vi "FTW-JSON-Core-GetFlattenedValue.vi"(0 "Library Filepath":path, 5 "JSON Element":i64 format="%016x", 7 "LabVIEW Type":T1, 9 "Element Default Value":variant, 11 "error in":errorcluster, 12 "Encoding Flags":i64 format="%016x") -> (4 "Flattened Value":string, 15 "error out":errorcluster)   [LabVIEW 2014, in "FTW-JSON-Fetch.xnode"]
uses:
  FTW-JSON-Fetch.xnode
  src/reflection/FTW-Reflection-Types.ctl
  src/json/core/FTW-JSON-Core-Type.ctl
  src/error/FTW-ERR-ThrowError.vi
  src/error/FTW-ERR-NoErrorConstant.vi
  src/error/FTW-ERR-CallChain.vi
  src/string/FTW-STR-ReplaceWhitespace.vi
panel:
  # "Inputs"
  # "Outputs"
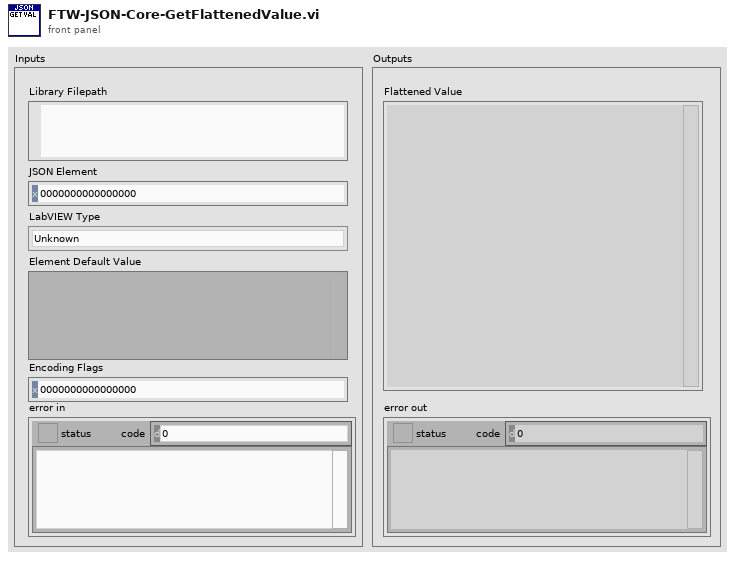
[diagram p1: front panel]
types:
  T1 = typedef "FTW-Reflection-Types.ctl" = enum16{"Unknown", "Void", "Array", "Cluster", "LVObject", "Boolean", "I8", "I16", "I32", "I64", "U8", "U16", "U32", "U64", "SGL", "DBL", "EXT", "CSG", "CDB", "CXT", "FXP", "EnumU8", "EnumU16", "EnumU32", "EnumU64", "SGLwithUnit", "DBLwithUnit", "EXTwithUnit", "CSGwithUnit", "CDBwithUnit", "CXTwithUnit", "String", "Path", "Picture", "Tag", "LVVariant", "Timestamp", "WaveformI8", "WaveformI16", "WaveformI32", "WaveformI64", "WaveformU8", "WaveformU16", "WaveformU32", "WaveformU64", "WaveformSGL", "WaveformDBL", "WaveformEXT", "WaveformCSG", "WaveformCDB", "WaveformCXT", "WaveformDigital", "WaveformUnknownType", "DigitalData", "DynamicData", "ExternalData", "FileByteStream", "TDMStream", "dotNET", "ActiveX", "VIServerReference", "VIReference", "ApplicationInstance", "Menu", "ConnectionDataSocket", "ConnectionVISA", "ConnectionBluetooth", "ConnectionIrDA", "ConnectionTCP", "ConnectionUDP", "ConnectionHTTPClient", "ConnectionFTP", "Occurrence", "Notifier", "Queue", "Rendezvous", "Semaphore", "RTFIFO", "EventPublisher", "EventRegistration", "EventCallback", "DataValueReference", "GenericClass", "GenericClassTag", "GenericClassDeepCopy", "GenericClassFlattened", "GenericClassTagFlattened", "GenericReferenceType", "WindowsRegistry", "OverloadedDatalogRef", "ReferenceUnknownType", "ByteArray"}
  T2 = typedef "FTW-JSON-Core-Type.ctl" = enum8{"Object", "Array", "String", "Integer", "Floating Point", "true", "false", "null", "undefined"}
  T3 = cluster{"Element Name":string, "Element Type":T1, "Element Value":variant}[]
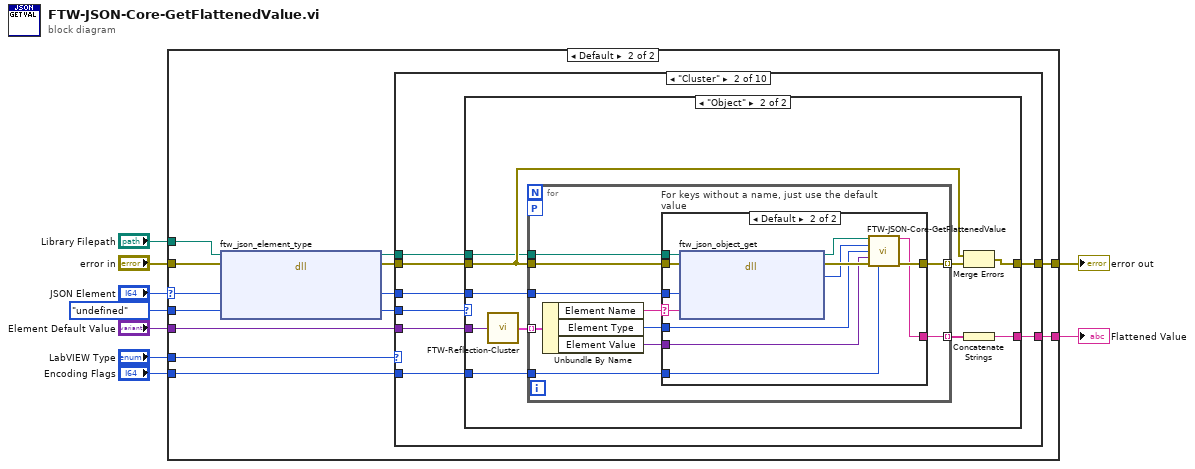
[diagram p0: block diagram]
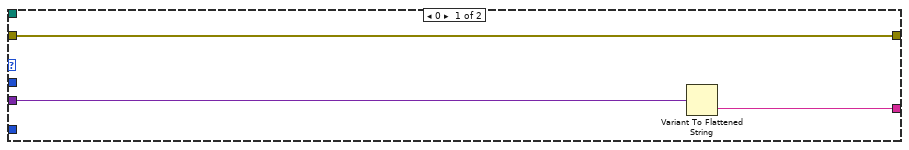
[diagram p2: hidden frame]
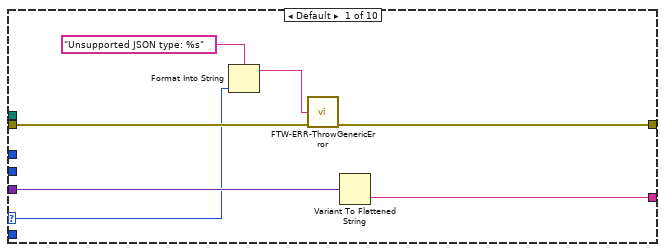
[diagram p3: hidden frame]
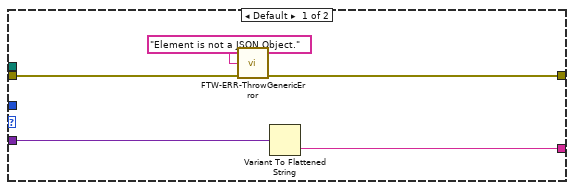
[diagram p4: hidden frame]
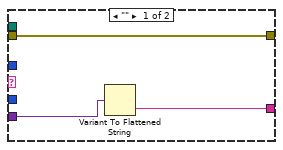
[diagram p5: hidden frame]
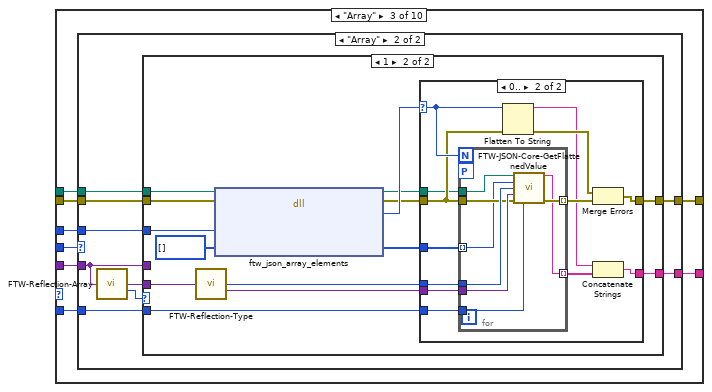
[diagram p6: hidden frame]
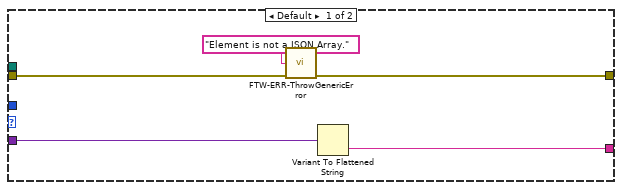
[diagram p7: hidden frame]
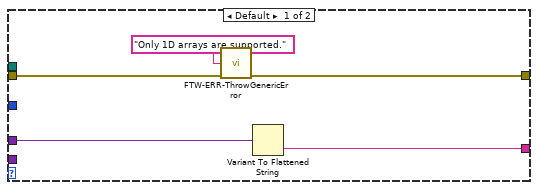
[diagram p8: hidden frame]
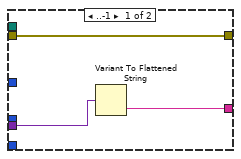
[diagram p9: hidden frame]
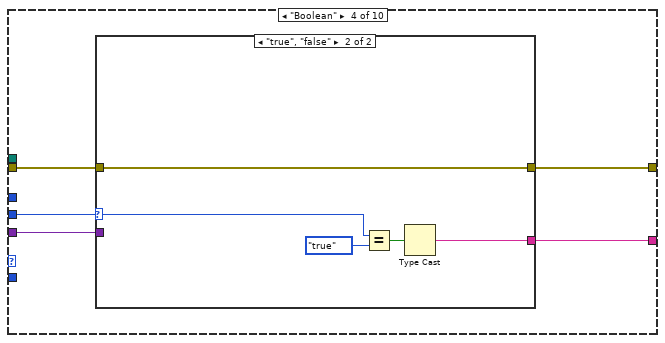
[diagram p10: hidden frame]
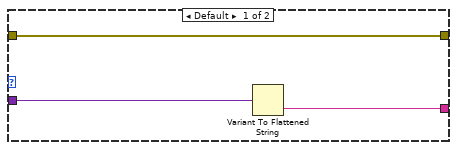
[diagram p11: hidden frame]
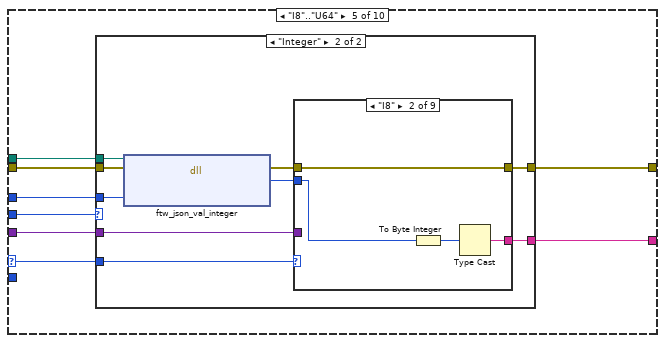
[diagram p12: hidden frame]
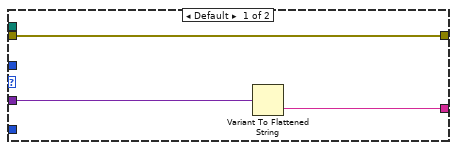
[diagram p13: hidden frame]
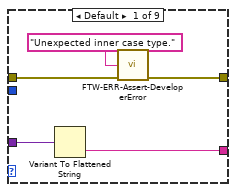
[diagram p14: hidden frame]
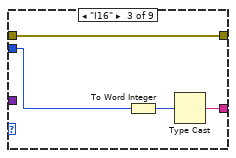
[diagram p15: hidden frame]
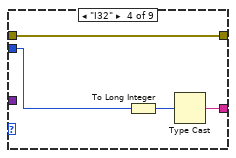
[diagram p16: hidden frame]
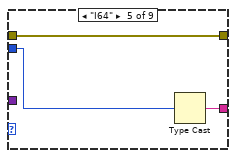
[diagram p17: hidden frame]
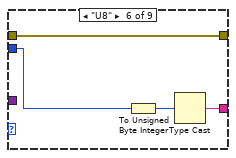
[diagram p18: hidden frame]
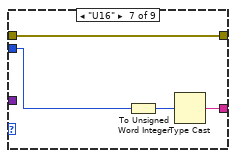
[diagram p19: hidden frame]
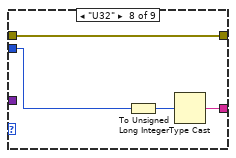
[diagram p20: hidden frame]
diagram:
  n1 = case shown="Default" "JSON Element" {
    selector: "JSON Element" -> [_ w20]
    tunnel: [w10 w25] -> w9
    tunnel: [w11 w24] -> w7
    tunnel: "LabVIEW Type" -> [_ w23]
    tunnel: "Element Default Value" -> [w12 w22]
    tunnel: "error in" -> [w10 w14]
    tunnel: "Encoding Flags" -> [_ w21]
    tunnel: FTW-JSON-Core-Type."undefined" ("x") -> [_ w18]
    tunnel: "Library Filepath" -> [_ w15]
    frame 0 {
      n2 = Variant To Flattened String(Variant=w12) -> (data string=w11:string)  [unwired: 1 out]
    }
    frame Default {
      n3 = dll-call lib="?" fn="ftw_json_element_type"(path in=w15, error in=w14, "JSON Element"=w20, "JSON Type"=w18) -> (path out=w13:path, error out=w16:errorcluster, "JSON Element"=w19:i64, "JSON Type"=w17:T2)  [unwired: 2 in]
      n4 = case shown="\"Cluster\"" w23 {
        selector: w23 -> [w26 _ _ _ w163 w219 w303 _ w379 _]
        tunnel: [w29 w37 w86 w146 w160 w216 w300 w358 w376 w428] -> w25
        tunnel: [w27 w39 w87 w149 w165 w221 w305 w362 w381 w432] -> w24
        tunnel: w16 -> [w30 w36 w85 w150 w166 w222 w306 w363 w382 w433]
        tunnel: w19 -> [_ w38 w83 _ w162 w218 w302 w360 w378 w430]
        tunnel: w22 -> [w28 w40 w88 w148 w164 w220 w304 w361 w380 w431]
        tunnel: w17 -> [_ w35 w84 w147 w161 w217 w301 w359 w377 w429]
        tunnel: w21 -> [_ w34 w82 _ _ _ _ _ w375 _]
        tunnel: w13 -> [_ w33 w81 _ w159 w215 w299 w357 w374 w427]
        frame Default {
          n5 = Format Into String(format string="Unsupported JSON type: %s", w26) -> (resulting string=w32:string)  [unwired: 2 in, 1 out]
          n6 = call "FTW-ERR-ThrowGenericError.vi"("Error Message"=w32, "error in"=w30) -> ("error out"=w29:errorcluster)  [unwired: 13 in]
          n7 = Variant To Flattened String(Variant=w28) -> (data string=w27:string)  [unwired: 1 out]
        }
        frame "Cluster" {
          n8 = case shown="\"Object\"" w35 {
            tunnel: w40 -> [w43 w55]
            tunnel: [w42 w54] -> w39
            tunnel: w38 -> [_ w47]
            tunnel: [w44 w53] -> w37
            tunnel: w36 -> [w45 w48]
            tunnel: w34 -> [_ w52]
            tunnel: w33 -> [_ w46]
            frame Default {
              n9 = call "FTW-ERR-ThrowGenericError.vi"("Error Message"="Element is not a JSON Object.", "error in"=w45) -> ("error out"=w44:errorcluster)  [unwired: 13 in]
              n10 = Variant To Flattened String(Variant=w43) -> (data string=w42:string)  [unwired: 1 out]
            }
            frame "Object" {
              n11 = call "FTW-Reflection-Cluster.vi"("Cluster"=w55) -> ("Cluster Elements"=w51:T3)  [unwired: 14 in]
              n12 = for {
                tunnel: w51 -> [w64] mode=indexing
                tunnel: [w62] -> w50 mode=indexing
                tunnel: w47 -> [w59]
                tunnel: w48 -> [w65]
                tunnel: [w60] -> w49 mode=indexing
                workers-P: _ -> [_]
                tunnel: w52 -> [w58]
                tunnel: w46 -> [w56]
                n13 = Unbundle By Name(w64) -> ("Element Name"=w57:string, "Element Type"=w61:T1, "Element Value"=w63:variant)
                n14 = case "For keys without a name, just use the default value" shown="Default" w57 {
                  selector: w57 -> [_ w77]
                  tunnel: w65 -> [w66 w79]
                  tunnel: w63 -> [w68 w74]
                  tunnel: [w67 w75] -> w62
                  tunnel: w59 -> [_ w78]
                  tunnel: w61 -> [_ w73]
                  tunnel: [w66 w76] -> w60
                  tunnel: w58 -> [_ w71]
                  tunnel: w56 -> [_ w70]
                  frame "" {
                    n15 = Variant To Flattened String(Variant=w68) -> (data string=w67:string)  [unwired: 1 out]
                  }
                  frame Default {
                    n16 = dll-call lib="?" fn="ftw_json_object_get"(path in=w70, error in=w79, "JSON Object Pointer"=w78, "Element Key"=w77) -> (path out=w69:path, error out=w80:errorcluster, "JSON Element Pointer"=w72:i64)  [unwired: 3 in]
                    n17 = call "FTW-JSON-Core-GetFlattenedValue.vi"("Library Filepath"=w69, "JSON Element"=w72, "LabVIEW Type"=w73, "Element Default Value"=w74, "error in"=w80, "Encoding Flags"=w71) -> ("Flattened Value"=w75:string, "error out"=w76:errorcluster)  [unwired: 8 in]
                  }
                }
              }
              n18 = Merge Errors(w48, w49) -> (w53:errorcluster)
              n19 = Concatenate Strings(w50) -> (w54:string)
            }
          }
        }
        frame "Array" {
          n20 = case shown="\"Array\"" w84 {
            tunnel: w88 -> [w91 w96]
            tunnel: [w90 w102] -> w87
            tunnel: [w89 w101] -> w86
            tunnel: w85 -> [w92 w100]
            tunnel: w83 -> [_ w97]
            tunnel: w82 -> [_ w95]
            tunnel: w81 -> [_ w94]
            frame Default {
              n21 = call "FTW-ERR-ThrowGenericError.vi"("Error Message"="Element is not a JSON Array.", "error in"=w92) -> ("error out"=w89:errorcluster)  [unwired: 13 in]
              n22 = Variant To Flattened String(Variant=w91) -> (data string=w90:string)  [unwired: 1 out]
            }
            frame "Array" {
              n23 = call "FTW-Reflection-Array.vi"("Array"=w96) -> ("Default Array Element"=w99:variant, "Number of Dimensions"=w98:i32)  [unwired: 13 in]
              n24 = case shown="1" w98 {
                tunnel: [w104 w121] -> w102
                tunnel: [w105 w120] -> w101
                tunnel: w100 -> [w106 w114]
                tunnel: w99 -> [_ w119]
                tunnel: w97 -> [_ w113]
                tunnel: w96 -> [w103 _]
                tunnel: w95 -> [_ w116]
                tunnel: w94 -> [_ w109]
                frame Default {
                  n25 = call "FTW-ERR-ThrowGenericError.vi"("Error Message"="Only 1D arrays are supported.", "error in"=w106) -> ("error out"=w105:errorcluster)  [unwired: 13 in]
                  n26 = Variant To Flattened String(Variant=w103) -> (data string=w104:string)  [unwired: 1 out]
                }
                frame 1 {
                  n27 = call "FTW-Reflection-Type.vi"("Anything"=w119) -> ("LabVIEW Type"=w118:T1, "Variant Type and Value"=w117:variant)  [unwired: 12 in, 1 out]
                  n28 = dll-call lib="?" fn="ftw_json_array_elements"(path in=w109, error in=w114, "Array Pointer"=w113, "Items"=i64[] []) -> (path out=w108:path, error out=w110:errorcluster, "Elements"=w112:i32, "Items"=w111:i64[])  [unwired: 2 in]
                  n29 = case shown="0.." w112 {
                    selector: w112 -> [_ w131]
                    tunnel: [w124 w137] -> w121
                    tunnel: [w122 w136] -> w120
                    tunnel: w110 -> [w122 w128]
                    tunnel: w118 -> [_ w134]
                    tunnel: w117 -> [w123 w133]
                    tunnel: w116 -> [_ w127]
                    tunnel: w111 -> [_ w126]
                    tunnel: w108 -> [_ w125]
                    frame ..-1 {
                      n30 = Variant To Flattened String(Variant=w123) -> (data string=w124:string)  [unwired: 1 out]
                    }
                    frame 0.. {
                      n31 = for {
                        N: w131 -> [_]
                        workers-P: _ -> [_]
                        tunnel: w128 -> [w140]
                        tunnel: [w145] -> w135 mode=indexing
                        tunnel: w134 -> [w142]
                        tunnel: w133 -> [w143]
                        tunnel: [w144] -> w132 mode=indexing
                        tunnel: w127 -> [w141]
                        tunnel: w126 -> [w139] mode=indexing
                        tunnel: w125 -> [w138]
                        n32 = call "FTW-JSON-Core-GetFlattenedValue.vi"("Library Filepath"=w138, "JSON Element"=w139, "LabVIEW Type"=w142, "Element Default Value"=w143, "error in"=w140, "Encoding Flags"=w141) -> ("Flattened Value"=w144:string, "error out"=w145:errorcluster)  [unwired: 8 in]
                      }
                      n33 = Flatten To String(anything=w131, error in (no error)=w128) -> (data string=w129:string, error out=w130:errorcluster)  [unwired: 2 in, 1 out]
                      n34 = Merge Errors(w130, w135) -> (w136:errorcluster)
                      n35 = Concatenate Strings(w129, w132) -> (w137:string)
                    }
                  }
                }
              }
            }
          }
        }
        frame "Boolean" {
          n36 = case shown="\"true\", \"false\"" w147 {
            selector: w147 -> [_ w156]
            tunnel: w150 -> [w151 w157]
            tunnel: w148 -> [w153 _]
            tunnel: [w152 w158] -> w149
            tunnel: [w151 w157] -> w146
            frame Default {
              n37 = Variant To Flattened String(Variant=w153) -> (data string=w152:string)  [unwired: 1 out]
            }
            frame "true", "false" {
              n38 = Equal?(x=w156, y=FTW-JSON-Core-Type."true" ("x")) -> (x = y?=w154:bool)
              n39 = Type Cast(x=w154) -> (*(type *) &x=w158:string)  [unwired: 1 in]
            }
          }
        }
        frame "I8".."U64" {
          n40 = case shown="\"Integer\"" w161 {
            tunnel: w162 -> [_ w178]
            tunnel: w166 -> [w167 w177]
            tunnel: w164 -> [w169 w171]
            tunnel: [w168 w172] -> w165
            tunnel: [w167 w175] -> w160
            tunnel: w163 -> [_ w176]
            tunnel: w159 -> [_ w170]
            frame Default {
              n41 = Variant To Flattened String(Variant=w169) -> (data string=w168:string)  [unwired: 1 out]
            }
            frame "Integer" {
              n42 = dll-call lib="?" fn="ftw_json_val_integer"(path in=w170, error in=w177, "JSON Element Pointer"=w178) -> (error out=w174:errorcluster, "I64 Value"=w173:i64)  [unwired: 2 in, 1 out]
              n43 = case shown="\"I8\"" w176 {
                tunnel: [w182 w187 w191 w195 w198 w202 w206 w210 w214] -> w175
                tunnel: w174 -> [w183 w187 w191 w195 w198 w202 w206 w210 w214]
                tunnel: w173 -> [_ w185 w189 w193 w196 w200 w204 w208 w212]
                tunnel: [w179 w186 w190 w194 w197 w201 w205 w209 w213] -> w172
                tunnel: w171 -> [w180 _ _ _ _ _ _ _ _]
                frame Default {
                  n44 = Variant To Flattened String(Variant=w180) -> (data string=w179:string)  [unwired: 1 out]
                  n45 = call "FTW-ERR-Assert-DeveloperError.vi"("Reason this error should never happen"="Unexpected inner case type.", "error in"=w183) -> ("error out"=w182:errorcluster)  [unwired: 13 in]
                }
                frame "I8" {
                  n46 = To Byte Integer(number=w185) -> (8bit integer=w184:i8)
                  n47 = Type Cast(x=w184) -> (*(type *) &x=w186:string)  [unwired: 1 in]
                }
                frame "I16" {
                  n48 = To Word Integer(number=w189) -> (16bit integer=w188:i16)
                  n49 = Type Cast(x=w188) -> (*(type *) &x=w190:string)  [unwired: 1 in]
                }
                frame "I32" {
                  n50 = To Long Integer(number=w193) -> (32bit integer=w192:i32)
                  n51 = Type Cast(x=w192) -> (*(type *) &x=w194:string)  [unwired: 1 in]
                }
                frame "I64" {
                  n52 = Type Cast(x=w196) -> (*(type *) &x=w197:string)  [unwired: 1 in]
                }
                frame "U8" {
                  n53 = To Unsigned Byte Integer(number=w200) -> (unsigned 8bit integer=w199:u8)
                  n54 = Type Cast(x=w199) -> (*(type *) &x=w201:string)  [unwired: 1 in]
                }
                frame "U16" {
                  n55 = To Unsigned Word Integer(number=w204) -> (unsigned 16bit integer=w203:u16)
                  n56 = Type Cast(x=w203) -> (*(type *) &x=w205:string)  [unwired: 1 in]
                }
                frame "U32" {
                  n57 = To Unsigned Long Integer(number=w208) -> (unsigned 32bit integer=w207:u32)
                  n58 = Type Cast(x=w207) -> (*(type *) &x=w209:string)  [unwired: 1 in]
                }
                frame "U64" {
                  n59 = To Unsigned Quad Integer(1:w212) -> (0:w211:u64)
                  n60 = Type Cast(x=w211) -> (*(type *) &x=w213:string)  [unwired: 1 in]
                }
              }
            }
          }
        }
        frame "EnumU8".."EnumU64" {
          n61 = case shown="\"Integer\"" w217 {
            tunnel: w218 -> [_ w235 w272]
            tunnel: w222 -> [w223 w234 w273]
            tunnel: w220 -> [w225 w229 w277]
            tunnel: [w224 w230 w274] -> w221
            tunnel: [w223 w232 w275] -> w216
            tunnel: w219 -> [_ w233 w276]
            tunnel: w215 -> [_ w226 w269]
            frame Default {
              n62 = Variant To Flattened String(Variant=w225) -> (data string=w224:string)  [unwired: 1 out]
            }
            frame "String" {
              n63 = dll-call lib="?" fn="ftw_json_val_string"(path in=w226, error in=w234, "JSON Element Pointer"=w235, "Value"="") -> (error out=w231:errorcluster, "Value"=w227:string)  [unwired: 3 in, 1 out]
              n64 = case shown="Default" w233 {
                tunnel: [w239 w247 w254 w261 w268] -> w232
                tunnel: w231 -> [w240 w247 w254 w261 w268]
                tunnel: w227 -> [_ w244 w251 w258 w265]
                tunnel: [w236 w243 w250 w257 w264] -> w230
                tunnel: w229 -> [w237 w246 w253 w260 w267]
                frame Default {
                  n65 = Variant To Flattened String(Variant=w237) -> (data string=w236:string)  [unwired: 1 out]
                  n66 = call "FTW-ERR-Assert-DeveloperError.vi"("Reason this error should never happen"="Unexpected inner case type.", "error in"=w240) -> ("error out"=w239:errorcluster)  [unwired: 13 in]
                }
                frame "EnumU8" {
                  n67 = call "FTW-Reflection-Enum.vi"("Enum"=w246) -> ("Enum Items"=w245:string[])  [unwired: 12 in, 2 out]
                  n68 = Search 1D Array(1D array=w245, element=w244) -> (index of element=w242:i32)  [unwired: 1 in]
                  n69 = To Unsigned Byte Integer(number=w242) -> (unsigned 8bit integer=w241:u8)
                  n70 = Type Cast(x=w241) -> (*(type *) &x=w243:string)  [unwired: 1 in]
                }
                frame "EnumU16" {
                  n71 = call "FTW-Reflection-Enum.vi"("Enum"=w253) -> ("Enum Items"=w252:string[])  [unwired: 12 in, 2 out]
                  n72 = Search 1D Array(1D array=w252, element=w251) -> (index of element=w249:i32)  [unwired: 1 in]
                  n73 = To Unsigned Word Integer(number=w249) -> (unsigned 16bit integer=w248:u16)
                  n74 = Type Cast(x=w248) -> (*(type *) &x=w250:string)  [unwired: 1 in]
                }
                frame "EnumU32" {
                  n75 = call "FTW-Reflection-Enum.vi"("Enum"=w260) -> ("Enum Items"=w259:string[])  [unwired: 12 in, 2 out]
                  n76 = Search 1D Array(1D array=w259, element=w258) -> (index of element=w256:i32)  [unwired: 1 in]
                  n77 = To Unsigned Long Integer(number=w256) -> (unsigned 32bit integer=w255:u32)
                  n78 = Type Cast(x=w255) -> (*(type *) &x=w257:string)  [unwired: 1 in]
                }
                frame "EnumU64" {
                  n79 = call "FTW-Reflection-Enum.vi"("Enum"=w267) -> ("Enum Items"=w266:string[])  [unwired: 12 in, 2 out]
                  n80 = Search 1D Array(1D array=w266, element=w265) -> (index of element=w263:i32)  [unwired: 1 in]
                  n81 = To Unsigned Quad Integer(1:w263) -> (0:w262:u64)
                  n82 = Type Cast(x=w262) -> (*(type *) &x=w264:string)  [unwired: 1 in]
                }
              }
            }
            frame "Integer" {
              n83 = dll-call lib="?" fn="ftw_json_val_integer"(path in=w269, error in=w273, "JSON Element Pointer"=w272) -> (error out=w270:errorcluster, "I64 Value"=w271:i64)  [unwired: 2 in, 1 out]
              n84 = case shown="\"EnumU8\"" w276 {
                tunnel: [w281 w286 w290 w294 w298] -> w275
                tunnel: w270 -> [w282 w286 w290 w294 w298]
                tunnel: w271 -> [_ w284 w288 w292 w296]
                tunnel: [w278 w285 w289 w293 w297] -> w274
                tunnel: w277 -> [w279 _ _ _ _]
                frame Default {
                  n85 = Variant To Flattened String(Variant=w279) -> (data string=w278:string)  [unwired: 1 out]
                  n86 = call "FTW-ERR-Assert-DeveloperError.vi"("Reason this error should never happen"="Unexpected inner case type.", "error in"=w282) -> ("error out"=w281:errorcluster)  [unwired: 13 in]
                }
                frame "EnumU8" {
                  n87 = To Unsigned Byte Integer(number=w284) -> (unsigned 8bit integer=w283:u8)
                  n88 = Type Cast(x=w283) -> (*(type *) &x=w285:string)  [unwired: 1 in]
                }
                frame "EnumU16" {
                  n89 = To Unsigned Word Integer(number=w288) -> (unsigned 16bit integer=w287:u16)
                  n90 = Type Cast(x=w287) -> (*(type *) &x=w289:string)  [unwired: 1 in]
                }
                frame "EnumU32" {
                  n91 = To Unsigned Long Integer(number=w292) -> (unsigned 32bit integer=w291:u32)
                  n92 = Type Cast(x=w291) -> (*(type *) &x=w293:string)  [unwired: 1 in]
                }
                frame "EnumU64" {
                  n93 = To Unsigned Quad Integer(1:w296) -> (0:w295:u64)
                  n94 = Type Cast(x=w295) -> (*(type *) &x=w297:string)  [unwired: 1 in]
                }
              }
            }
          }
        }
        frame "SGL".."EXT" {
          n95 = case shown="\"Integer\", \"Floating Point\"" w301 {
            tunnel: w302 -> [_ w314 _]
            tunnel: w306 -> [w307 w312 w336]
            tunnel: w304 -> [w309 w315 w337]
            tunnel: [w308 w316 w338] -> w305
            tunnel: [w307 w317 w339] -> w300
            tunnel: w303 -> [_ w318 w340]
            tunnel: w299 -> [_ w310 _]
            frame Default {
              n96 = Variant To Flattened String(Variant=w309) -> (data string=w308:string)  [unwired: 1 out]
            }
            frame "Integer", "Floating Point" {
              n97 = dll-call lib="?" fn="ftw_json_val_double"(path in=w310, error in=w312, "JSON Element Pointer"=w314) -> (error out=w311:errorcluster, "DBL Value"=w313:dbl)  [unwired: 2 in, 1 out]
              n98 = case shown="\"SGL\"" w318 {
                tunnel: [w322 w327 w330 w334] -> w317
                tunnel: w311 -> [w323 w327 w330 w334]
                tunnel: w313 -> [_ w324 w328 w332]
                tunnel: [w319 w326 w329 w333] -> w316
                tunnel: w315 -> [w320 _ _ _]
                frame Default {
                  n99 = Variant To Flattened String(Variant=w320) -> (data string=w319:string)  [unwired: 1 out]
                  n100 = call "FTW-ERR-Assert-DeveloperError.vi"("Reason this error should never happen"="Unexpected inner case type.", "error in"=w323) -> ("error out"=w322:errorcluster)  [unwired: 13 in]
                }
                frame "SGL" {
                  n101 = To Single Precision Float(number=w324) -> (single precision float=w325:sgl)
                  n102 = Type Cast(x=w325) -> (*(type *) &x=w326:string)  [unwired: 1 in]
                }
                frame "DBL" {
                  n103 = Type Cast(x=w328) -> (*(type *) &x=w329:string)  [unwired: 1 in]
                }
                frame "EXT" {
                  n104 = To Extended Precision Float(1:w332) -> (0:w331:ext)
                  n105 = Type Cast(x=w331) -> (*(type *) &x=w333:string)  [unwired: 1 in]
                }
              }
            }
            frame "null" {
              n106 = case shown="\"SGL\"" w340 {
                tunnel: [w344 w349 w352 w356] -> w339
                tunnel: w336 -> [w345 w349 w352 w356]
                tunnel: nan ("DBL Value") -> [_ w346 w350 w354]
                tunnel: [w341 w348 w351 w355] -> w338
                tunnel: w337 -> [w342 _ _ _]
                frame Default {
                  n107 = Variant To Flattened String(Variant=w342) -> (data string=w341:string)  [unwired: 1 out]
                  n108 = call "FTW-ERR-Assert-DeveloperError.vi"("Reason this error should never happen"="Unexpected inner case type.", "error in"=w345) -> ("error out"=w344:errorcluster)  [unwired: 13 in]
                }
                frame "SGL" {
                  n109 = To Single Precision Float(number=w346) -> (single precision float=w347:sgl)
                  n110 = Type Cast(x=w347) -> (*(type *) &x=w348:string)  [unwired: 1 in]
                }
                frame "DBL" {
                  n111 = Type Cast(x=w350) -> (*(type *) &x=w351:string)  [unwired: 1 in]
                }
                frame "EXT" {
                  n112 = To Extended Precision Float(1:w354) -> (0:w353:ext)
                  n113 = Type Cast(x=w353) -> (*(type *) &x=w355:string)  [unwired: 1 in]
                }
              }
            }
          }
        }
        frame "Timestamp" {
          n114 = case shown="\"Floating Point\"" w359 {
            tunnel: w360 -> [_ w371]
            tunnel: w363 -> [w364 w368]
            tunnel: w361 -> [w366 _]
            tunnel: [w365 w373] -> w362
            tunnel: [w364 w369] -> w358
            tunnel: w357 -> [_ w367]
            frame Default {
              n115 = Variant To Flattened String(Variant=w366) -> (data string=w365:string)  [unwired: 1 out]
            }
            frame "Floating Point" {
              n116 = dll-call lib="?" fn="ftw_json_val_double"(path in=w367, error in=w368, "JSON Element Pointer"=w371) -> (error out=w369:errorcluster, "DBL Value"=w370:dbl)  [unwired: 2 in, 1 out]
              n117 = To Time Stamp(1:w370) -> (0:w372:timestamp)
              n118 = Type Cast(x=w372) -> (*(type *) &x=w373:string)  [unwired: 1 in]
            }
          }
        }
        frame "String".."Picture", "ConnectionVISA" {
          n119 = case shown="\"String\"" w377 {
            tunnel: w378 -> [w388 _ w400]
            tunnel: w382 -> [w386 w392 w398]
            tunnel: w380 -> [_ w394 w401]
            tunnel: [w391 w393 w402] -> w381
            tunnel: [w390 w392 w403] -> w376
            tunnel: w379 -> [_ _ w404]
            tunnel: w375 -> [w387 _ _]
            tunnel: w374 -> [w383 _ w395]
            frame Default {
              n120 = dll-call lib="?" fn="ftw_json_serialize_element"(path in=w383, error in=w386, "JSON Object Pointer"=w388, "Flags"=w387, "Serialized String"="") -> (error out=w385:errorcluster, "Serialized String"=w384:string)  [unwired: 4 in, 1 out]
              n121 = Flatten To String(anything=w384, error in (no error)=w385) -> (data string=w391:string, error out=w390:errorcluster)  [unwired: 2 in, 1 out]
            }
            frame "undefined" {
              n122 = Variant To Flattened String(Variant=w394) -> (data string=w393:string)  [unwired: 1 out]
            }
            frame "String" {
              n123 = dll-call lib="?" fn="ftw_json_val_string"(path in=w395, error in=w398, "JSON Element Pointer"=w400, "Value"="") -> (error out=w399:errorcluster, "Value"=w397:string)  [unwired: 3 in, 1 out]
              n124 = case shown="\"ConnectionVISA\"" w404 {
                tunnel: [w408 w412 w416 w421 w426] -> w403
                tunnel: w399 -> [w409 w413 w417 w422 w426]
                tunnel: w397 -> [_ w411 w415 w420 w425]
                tunnel: [w405 w410 w414 w419 w424] -> w402
                tunnel: w401 -> [w406 _ _ _ _]
                frame Default {
                  n125 = Variant To Flattened String(Variant=w406) -> (data string=w405:string)  [unwired: 1 out]
                  n126 = call "FTW-ERR-Assert-DeveloperError.vi"("Reason this error should never happen"="Unexpected inner case type.", "error in"=w409) -> ("error out"=w408:errorcluster)  [unwired: 13 in]
                }
                frame "String" {
                  n127 = Flatten To String(anything=w411, error in (no error)=w413) -> (data string=w410:string, error out=w412:errorcluster)  [unwired: 2 in, 1 out]
                }
                frame "ConnectionVISA" {
                  n128 = Flatten To String(anything=w415, error in (no error)=w417) -> (data string=w414:string, error out=w416:errorcluster)  [unwired: 2 in, 1 out]
                }
                frame "Path" {
                  n129 = String To Path(string=w420) -> (path=w418:path)
                  n130 = Flatten To String(anything=w418, error in (no error)=w422) -> (data string=w419:string, error out=w421:errorcluster)  [unwired: 2 in, 1 out]
                }
                frame "Picture" {
                  n131 = call "FTW-STR-Encode-Base64.vi"("Input"=w425, "Direction"=enum16{"Encode", "Decode"}."Decode") -> ("Output"=w424:string)
                }
              }
            }
          }
        }
        frame "FileByteStream".."ConnectionDataSocket", "ConnectionBluetooth".."ReferenceUnknownType" {
          n132 = case shown="\"String\"" w429 {
            tunnel: w430 -> [_ w442]
            tunnel: w433 -> [w434 w443]
            tunnel: w431 -> [w436 w446]
            tunnel: [w435 w448] -> w432
            tunnel: [w434 w444] -> w428
            tunnel: w427 -> [_ w437]
            frame Default {
              n133 = Variant To Flattened String(Variant=w436) -> (data string=w435:string)  [unwired: 1 out]
            }
            frame "String" {
              w449 = "0x%16x"  # Reference Format
              n134 = dll-call lib="?" fn="ftw_json_val_string"(path in=w437, error in=w443, "JSON Element Pointer"=w442, "Value"="") -> (error out=w439:errorcluster, "Value"=w441:string)  [unwired: 3 in, 1 out]
              n135 = Scan From String(format string=w449, input string=w441, error in=w439, default 1=i64 0 ("default value 1")) -> (error out=w445:errorcluster, output 1=w447:i64)  [unwired: 1 in, 2 out]
              n136 = case shown="No Error" w445 {
                selector: w445 -> [w450 _]
                tunnel: [w454 w457] -> w448
                tunnel: w447 -> [w453 _]
                tunnel: w446 -> [_ w458]
                tunnel: [w450 w456] -> w444
                frame No Error {
                  n137 = Type Cast(type=refnum<k0> refnum, x=w453) -> (*(type *) &x=w452:refnum<k0>)
                  n138 = Type Cast(x=w452) -> (*(type *) &x=w454:string)  [unwired: 1 in]
                }
                frame Error {
                  n139 = Variant To Flattened String(Variant=w458) -> (data string=w457:string)  [unwired: 1 out]
                  n140 = call "FTW-ERR-ThrowGenericError.vi"("Error Message"="Unexpected reference format.") -> ("error out"=w456:errorcluster)  [unwired: 14 in]
                }
              }
            }
          }
        }
      }
    }
  }
  "error out" <- w9
  "Flattened Value" <- w7
